vi "Draw_Shape_Reangle.vi"(6 "Color":u32(colorbox)=16711680, 8 "error in":errorcluster, 10 "Rectangle Descriptor":T1, 11 "Image":T2) -> (0 "error out":errorcluster, 3 "Image Out":T2)   [LabVIEW 2019]
uses:
  <vilib>/vision/Image Controls.llb/IMAQ Image.ctl
panel:
  in  "Group":string
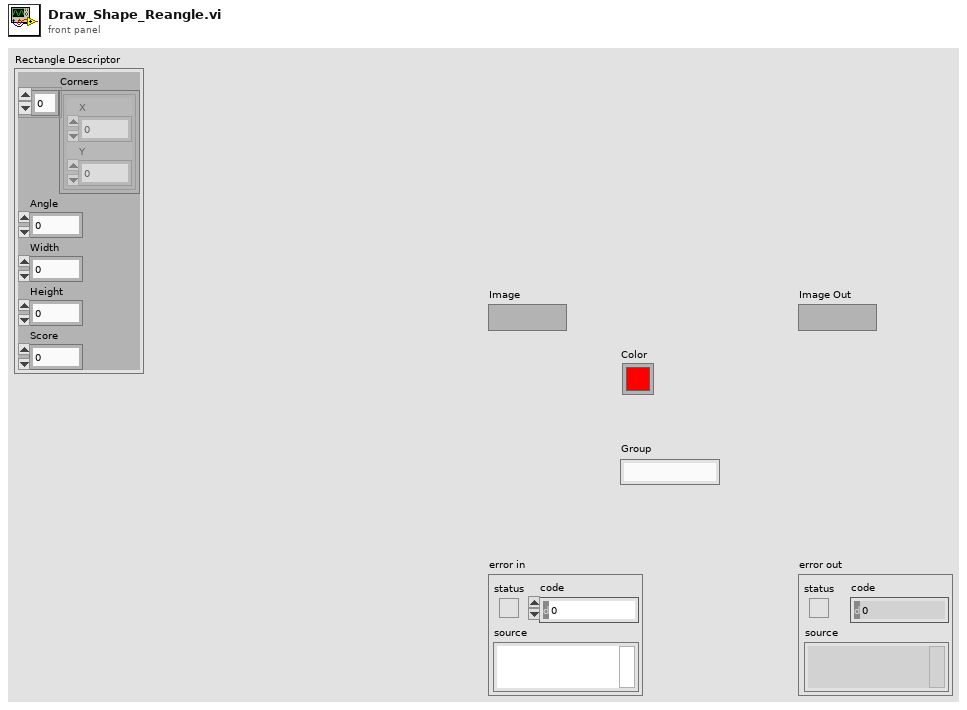
[diagram p1: front panel]
types:
  T1 = cluster{"Corners":cluster{"X":sgl, "Y":sgl}[], "Angle":dbl, "Width":dbl, "Height":dbl, "Score":dbl}
  T2 = typedef "IMAQ Image.ctl" = refnum<image>
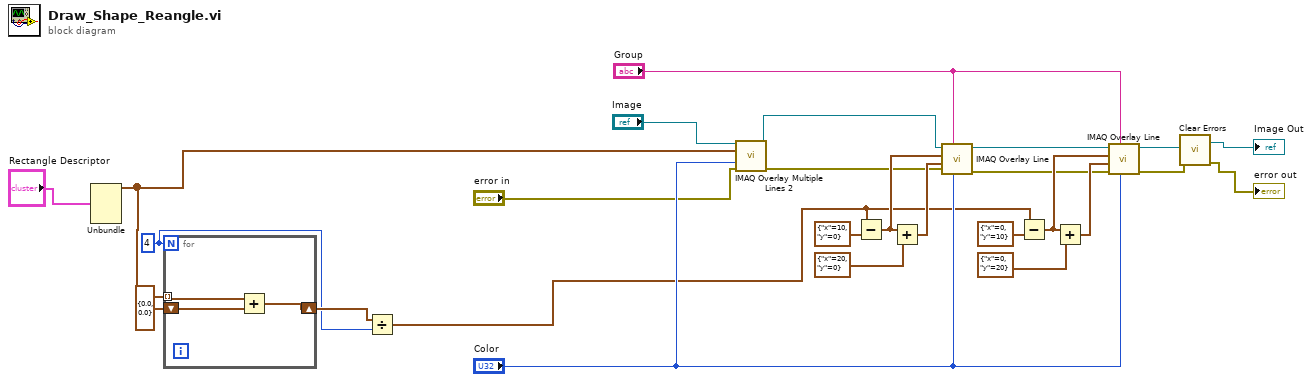
[diagram p0: block diagram]
diagram:
  w3 = 4
  n1 = Unbundle("Rectangle Descriptor") -> ("Corners"=w6:cluster{"X":sgl, "Y":sgl}[])  [unwired: 4 out]
  n2 = for {
    N: w3 -> [_]
    tunnel: w6 -> [w28] mode=indexing
    shift-right: [w26] -> w4
    shift-left: cluster{"X":sgl, "Y":sgl} {"X"=0.0, "Y"=0.0} -> [w27]
    n3 = Add(x=w28, y=w27) -> (x+y=w26:cluster{"X":sgl, "Y":sgl})
  }
  n4 = Divide(x=w4, y=w3) -> (x/y=w2:cluster{"X":sgl, "Y":sgl})
  n5 = call "IMAQ Overlay Multiple Lines 2"("Image"="Image", "Line End Points"=w6, "Color"="Color", "error in (no error)"="error in") -> ("Image Out"=w11:T2, "error out"=w8:errorcluster)  [unwired: 10 in]
  n6 = Subtract(x=w2, y=cluster{"x":i32, "y":i32} {"x"=10, "y"=0}) -> (x-y=w23:cluster{sgl, sgl})
  n7 = Add(x=w23, y=cluster{"x":i32, "y":i32} {"x"=20, "y"=0}) -> (x+y=w21:cluster{sgl, sgl})
  n8 = call "IMAQ Overlay Line"("Color"="Color", "Group"="Group", "error in (no error)"=w8, "End Point"=w21, "Start Point"=w23, "Image"=w11) -> ("error out"=w15:errorcluster, "Image Out"=w16:T2)  [unwired: 4 out]
  n9 = Subtract(x=w2, y=cluster{"x":i32, "y":i32} {"x"=0, "y"=10}) -> (x-y=w19:cluster{sgl, sgl})
  n10 = Add(x=w19, y=cluster{"x":i32, "y":i32} {"x"=0, "y"=20}) -> (x+y=w20:cluster{sgl, sgl})
  n11 = call "IMAQ Overlay Line"("Color"="Color", "Group"="Group", "error in (no error)"=w15, "End Point"=w20, "Start Point"=w19, "Image"=w16) -> ("error out"=w13:errorcluster, "Image Out"=→"Image Out":T2)  [unwired: 4 out]
  n12 = call <vilib>:"Clear Errors.vi"("error in (no error)"=w13) -> ("error out"=→"error out":errorcluster)  [unwired: 5 in, 1 out]
